vi "Offset_Loop_TS.vi"(0 "Port":u16, 1 "LV_Variables":T1={"ACQPS"=25, "Config_Enable"=1, "Prescale"=1, "ADC"=enum."A", "Adc_Channel"=1, "Ref_Int/EXT"=FALSE}, 2 "ACQPS":u16[](array[numeric]), 5 "Core":u16, 7 "Pin_Config":i32, 11 "error in":errorcluster, 12 "Voltage":dbl[](array[numeric]), 14 "VREF_Measured":dbl=2.5 format="%#_13g") -> (4 "Port Number out":u16, 6 "Core Number out":u16, 8 "output array":string[][](array[string]), 13 "OFF+GAIN":string[][](array[string]), 15 "error out":errorcluster)   [LabVIEW 2019]
uses:
  ADC_LV_Variables.ctl
  ADC_CTRL.ctl
  <userlib>/_TI-LA/Reusable/CCS/APIs/Data/Polymorphics/Write Data To Symbol - U16.vi
  <userlib>/_TI-LA/Reusable/CCS/APIs/CCS.lvlib
  <vilib>/Analysis/NI_AALBase.lvlib
  <userlib>/_TI-LA/Instr Drivers/Multimeter/Agilent 3446X Series/Agilent 3446X Series.lvlib
panel:
  out "AVG":dbl format="%0.2f"
  out "Array":dbl[](array[numeric])
  out "LV_Variables_out":T1={"ACQPS"=25, "Config_Enable"=1, "Prescale"=1, "ADC"=enum."A", "Adc_Channel"=1, "Ref_Int/EXT"=FALSE}
  in  "VISA_SGEN":refnum<visa-resource-name>="USB0::0x0957::0x1607::MY50001293::INSTR"
  out "standard deviation":dbl format="%0.2f"
  out "mean":dbl format="%0.2f"
  out "Waveform Graph":u16[](graph)
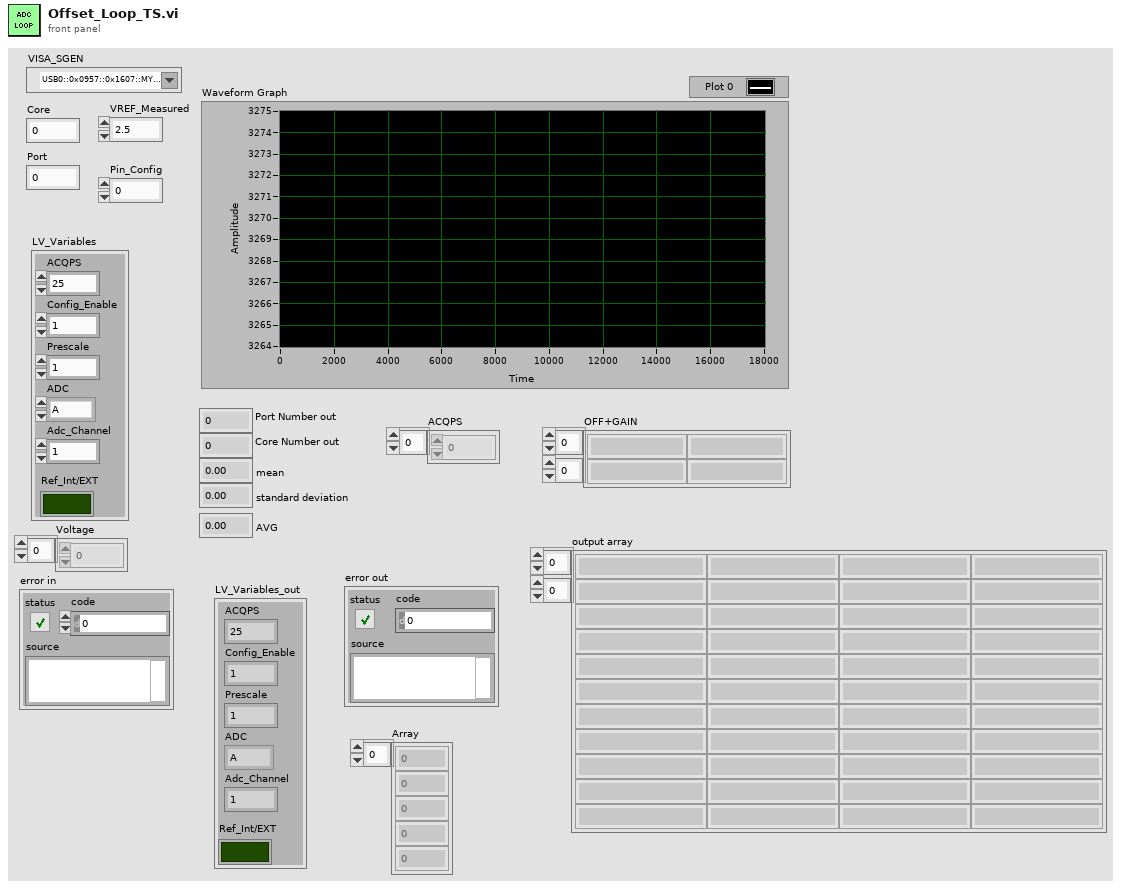
[diagram p1: front panel]
types:
  T1 = typedef "ADC_LV_Variables.ctl" = cluster{"ACQPS":u16, "Config_Enable":u16, "Prescale":u16, "ADC":T2, "Adc_Channel":u16, "Ref_Int/EXT":bool}
  T2 = typedef "ADC_CTRL.ctl" = enum16{"A", "B", "C"}
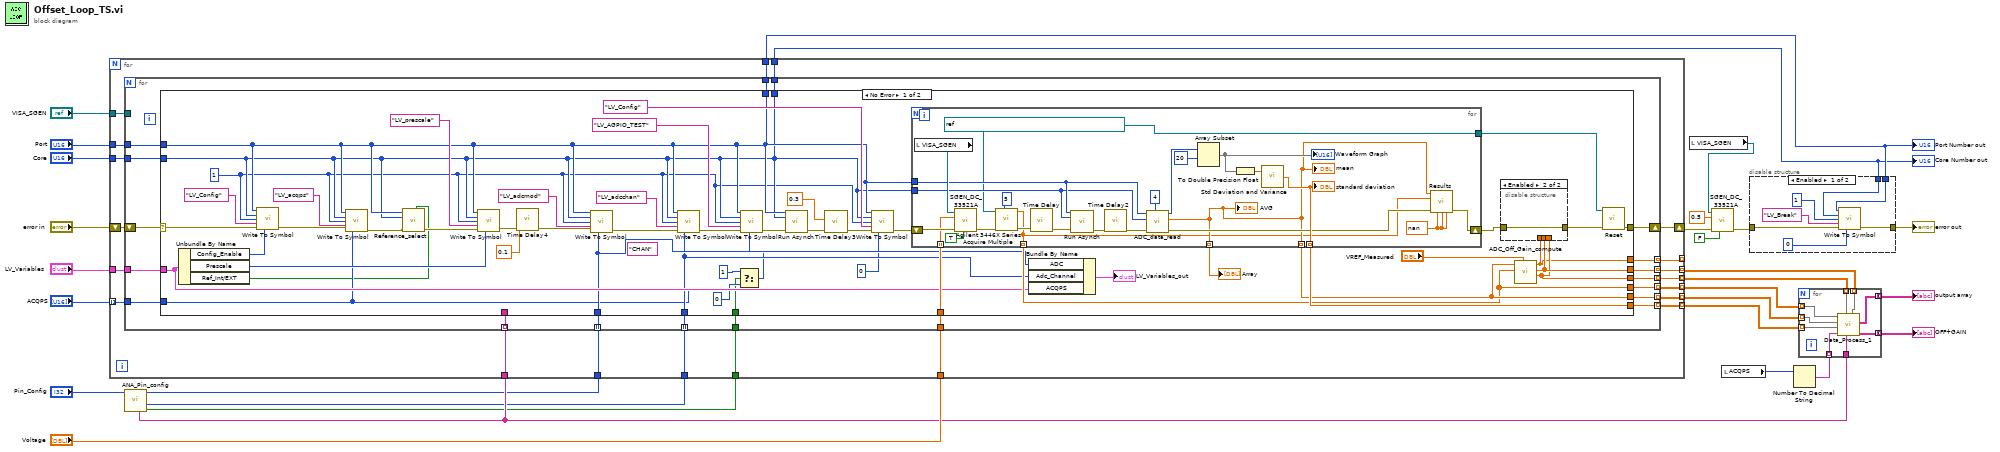
[diagram p0: block diagram]
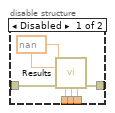
[diagram p3: hidden frame]
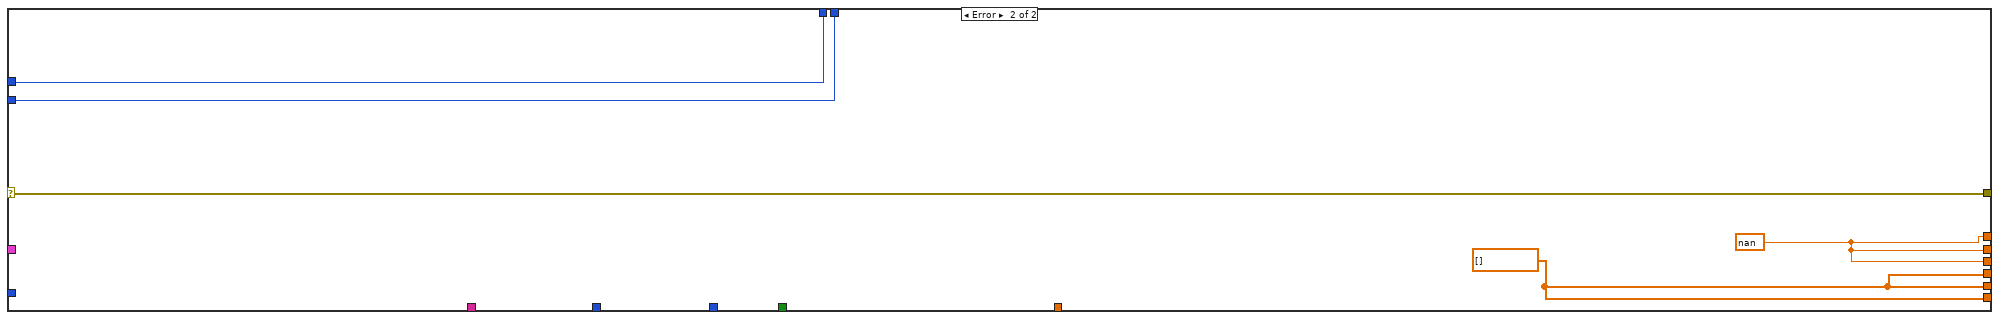
[diagram p4: hidden frame]
diagram:
  n1 = call "ANA_Pin_config.vi"("Pin_Config"="Pin_Config") -> ("Boolean"=w8:bool, "ADC_Channel"=w1:u16[], "ADC"=w2:T2[], "ADC+CH"=w9:string[])  [unwired: 7 in]
  n2 = for {
    tunnel: "Port" -> [w49]
    tunnel: "Core" -> [w48]
    tunnel: "LV_Variables" -> [w47]
    tunnel: [w45] -> w24
    tunnel: [w44] -> w23
    tunnel: w2 -> [w43]
    tunnel: w1 -> [w42]
    tunnel: "VISA_SGEN" -> [w41]
    tunnel: [w40] -> w10 mode=indexing
    tunnel: "Voltage" -> [w39]
    tunnel: [w38] -> w11 mode=indexing
    tunnel: [w37] -> w19 mode=indexing
    tunnel: [w36] -> w18 mode=indexing
    tunnel: [w35] -> w17 mode=indexing
    shift-right: [w46] -> w7
    shift-left: "error in" -> [w32]
    tunnel: "ACQPS" -> [w34] mode=indexing
    tunnel: w9 -> [w33]
    tunnel: w8 -> [w31]
    tunnel: [w30] -> _ mode=indexing
    n3 = for {
      tunnel: w49 -> [w65]
      tunnel: w48 -> [w66]
      tunnel: w47 -> [w67]
      shift-right: [w68] -> w46
      shift-left: w32 -> [w62]
      tunnel: [w63] -> w44
      tunnel: [w64] -> w45
      tunnel: w43 -> [w54] mode=indexing
      tunnel: w42 -> [w61] mode=indexing
      tunnel: [w60] -> w36 mode=indexing
      tunnel: [w59] -> w35 mode=indexing
      tunnel: w39 -> [w58]
      tunnel: w41 -> [_]
      tunnel: [w57] -> w40 mode=indexing
      tunnel: [w56] -> w38 mode=indexing
      tunnel: [w55] -> w37 mode=indexing
      tunnel: w34 -> [w53]
      tunnel: w33 -> [w52] mode=indexing
      tunnel: w31 -> [w51]
      tunnel: [w50] -> w30 mode=indexing
      n4 = case shown="No Error" w62 {
        selector: w62 -> [w111 w152]
        tunnel: [w92 w152] -> w68
        tunnel: w67 -> [w105 _]
        tunnel: w65 -> [w79 w154]
        tunnel: w66 -> [w78 w153]
        tunnel: [w79 w154] -> w64
        tunnel: [w78 w153] -> w63
        tunnel: w61 -> [w102 _]
        tunnel: [w109 w151] -> w60
        tunnel: [w110 w151] -> w59
        tunnel: w58 -> [w108 _]
        tunnel: [w89 w150] -> w57
        tunnel: [w88 w150] -> w56
        tunnel: [w107 w151] -> w55
        tunnel: w54 -> [w103 _]
        tunnel: w53 -> [w72 _]
        tunnel: w52 -> [_ _]
        tunnel: w51 -> [w95 _]
        tunnel: [w70 w150] -> w50
        frame No Error {
          (unwired) "CHAN" ("Name")
          w77 = 1 ("Page")
          n5 = Unbundle By Name(w105) -> ("Config_Enable"=w114:u16, "Prescale"=w106:u16, "Ref_Int/EXT"=w69:bool)
          n6 = call-poly <userlib>:"Write To Symbol.vi"("Port Number"=w79, "Core Number"=w78, "Page"=w77, "Symbol Name"="LV_Config", "error in"=w111, "Write Data"=w114) -> ("error out"=w118:errorcluster)  [unwired: 7 in, 2 out]
          n7 = call-poly <userlib>:"Write To Symbol.vi"("Port Number"=w79, "Core Number"=w78, "Page"=w77, "Symbol Name"="LV_acqps", "error in"=w118, "Write Data"=w72) -> ("error out"=w94:errorcluster)  [unwired: 7 in, 2 out]
          n8 = call "Reference_select.vi"("Internal_Ref"=w69, "error in"=w94, "Core Number"=w78, "Port Number"=w79) -> ("error out"=w93:errorcluster)  [unwired: 7 in]
          n9 = call-poly <userlib>:"Write To Symbol.vi"("Port Number"=w79, "Core Number"=w78, "Page"=w77, "Symbol Name"="LV_prescale", "error in"=w93, "Write Data"=w106) -> ("error out"=w76:errorcluster)  [unwired: 7 in, 2 out]
          n10 = call "Time Delay4"("error in (no error)"=w76, "Delay Time (s)"=0.1) -> ("error out"=w75:errorcluster)  [unwired: 9 in]
          n11 = call-poly <userlib>:"Write To Symbol.vi"("Port Number"=w79, "Core Number"=w78, "Page"=w77, "Symbol Name"="LV_adcmod", "error in"=w75, "Write Data"=w103) -> ("error out"=w101:errorcluster)  [unwired: 7 in, 2 out]
          n12 = call-poly <userlib>:"Write To Symbol.vi"("Port Number"=w79, "Core Number"=w78, "Page"=w77, "Symbol Name"="LV_adcchan", "error in"=w101, "Write Data"=w102) -> ("error out"=w100:errorcluster)  [unwired: 7 in, 2 out]
          n13 = Select(t=u16 1, s=w95, f=u16 0) -> (s? t:f=w98:u16)
          n14 = call-poly <userlib>:"Write To Symbol.vi"("Port Number"=w79, "Core Number"=w78, "Page"=w77, "Symbol Name"="LV_AGPIO_TEST", "error in"=w100, "Write Data"=w98) -> ("error out"=w85:errorcluster)  [unwired: 7 in, 2 out]
          n15 = call <userlib>:"Run Asynch.vi"("Port Number"=w79, "Core Number"=w78, "error in"=w85) -> ("error out"=w73:errorcluster)  [unwired: 10 in, 2 out]
          n16 = call "Time Delay3"("error in (no error)"=w73, "Delay Time (s)"=0.3) -> ("error out"=w83:errorcluster)  [unwired: 9 in]
          n17 = call-poly <userlib>:"Write To Symbol.vi"("Port Number"=w79, "Core Number"=w78, "Page"=w77, "Symbol Name"="LV_Config", "error in"=w83, "Write Data"=u16 0) -> ("error out"=w82:errorcluster)  [unwired: 7 in, 2 out]
          n18 = for {
            tunnel: w79 -> [w138]
            tunnel: w78 -> [w137]
            tunnel: [w127] -> w109 mode=indexing
            tunnel: [w144] -> w110 mode=indexing
            shift-right: [w130] -> w90
            shift-left: w82 -> [w141]
            tunnel: w108 -> [w136] mode=indexing
            tunnel: [w126] -> w107 mode=indexing
            tunnel: [w132] -> w91
            tunnel: [w127] -> w87 mode=indexing
            w129 = nan
            w132 = refnum<visa-resource-name> "USB0::0x2A8D::0x1301::MY57222838::INSTR" ("VISA resource name")
            n19 = local read "VISA_SGEN"() -> (w143:refnum<visa-resource-name>)
            n20 = call "SGEN_DC_33521A.vi"("Enable Output (T: Enable)"=TRUE, "error in (no error)"=w141, "DC Offset (0 V)"=w136, "VISA_SGEN"=w143) -> ("error out"=w135:errorcluster)  [unwired: 7 in]
            n21 = call "Agilent 3446X Series Acquire Multiple.vi"("Sample Count (1)"=5, "error in (no error)"=w135, "VISA resource name"=w132) -> ("error out"=w134:errorcluster, "mean"=w126:dbl)  [unwired: 6 in, 1 out]
            n22 = call "Time Delay"("error in (no error)"=w134) -> ("error out"=w142:errorcluster)  [unwired: 10 in]
            n23 = call <userlib>:"Run Asynch.vi"("Port Number"=w138, "Core Number"=w137, "error in"=w142) -> ("error out"=w140:errorcluster)  [unwired: 10 in, 2 out]
            n24 = call "Time Delay2"("error in (no error)"=w140) -> ("error out"=w139:errorcluster)  [unwired: 10 in]
            n25 = call "ADC_data_read.vi"("No_Iterations"=4, "error in (no error)"=w139, "Core Number"=w137, "Port Number"=w138) -> ("error out"=w131:errorcluster, "Read Data"=w127:dbl, "Read Data[]"=w146:u16[])  [unwired: 5 in]
            "mean" <- w127
            "AVG" <- w127
            n26 = Array Subset(array=w146, index=20) -> (w145:u16[])  [unwired: 1 in]
            "Waveform Graph" <- w145
            n27 = To Double Precision Float(number=w145) -> (double precision float=w148:dbl[])
            n28 = call <vilib>:"Std Deviation and Variance.vi"("X"=w148) -> ("standard deviation"=w144:dbl)  [unwired: 1 in, 2 out]
            "standard deviation" <- w144
            n29 = call "Results.vi"("Code"=w127, "Voltage"=w126, "Error In"=w131, "Slope"=w129, "Offset_Error"=w129, "Gain_error"=w129) -> ("error out"=w130:errorcluster)  [unwired: 9 in]
          }
          "Array" <- w87
          n30 = Bundle By Name(cluster=w105, "ADC"=w103, "Adc_Channel"=w102, "ACQPS"=w72) -> (→"LV_Variables_out":T1)
          n31 = call "ADC_Off_Gain_compute.vi"("VREF_Measured"="VREF_Measured", "Voltage_Array"=w107, "Code"=w109) -> ("Gain_Error_(LSB)"=w88:dbl, "Offset_Error"=w89:dbl, "slope"=w70:dbl)  [unwired: 5 in, 1 out]
          n32 = disable-structure shown="Enabled" {
            disable-tunnel: w90 -> [w124 w125]
            disable-tunnel: w70 -> [w122 _]
            disable-tunnel: w89 -> [w121 _]
            disable-tunnel: w88 -> [w120 _]
            disable-tunnel: [w119 w125] -> w71
            frame Disabled {
              w123 = nan
              n33 = call "Results.vi"("Code"=w123, "Voltage"=w123, "Error In"=w124, "Slope"=w122, "Offset_Error"=w121, "Gain_error"=w120) -> ("error out"=w119:errorcluster)  [unwired: 9 in]
            }
            frame Enabled {
            }
          }
          n34 = call <userlib>:"Reset.vi"("error in (no error)"=w71, "VISA resource name"=w91) -> ("error out"=w92:errorcluster)  [unwired: 8 in, 1 out]
        }
        frame Error {
          w150 = nan
          w151 = dbl[] []
        }
      }
    }
  }
  "Core Number out" <- w23
  "Port Number out" <- w24
  n35 = local read "VISA_SGEN"() -> (w5:refnum<visa-resource-name>)
  n36 = call "SGEN_DC_33521A.vi"("Enable Output (T: Enable)"=FALSE, "error in (no error)"=w7, "DC Offset (0 V)"=0.5, "VISA_SGEN"=w5) -> ("error out"=w6:errorcluster)  [unwired: 7 in]
  n37 = local read "ACQPS"() -> (w14:u16[])
  n38 = disable-structure shown="Enabled" {
    disable-tunnel: w6 -> [w158 w162]
    disable-tunnel: [w155 w162] -> w25
    disable-tunnel: w24 -> [w157 _]
    disable-tunnel: w23 -> [w156 _]
    frame Enabled {
      n39 = call-poly <userlib>:"Write To Symbol.vi"("Port Number"=w157, "Core Number"=w156, "Page"=1, "Symbol Name"="LV_Break", "error in"=w158, "Write Data"=u16 0) -> ("error out"=w155:errorcluster)  [unwired: 7 in, 2 out]
    }
    frame Disabled {
    }
  }
  "error out" <- w25
  n40 = Number To Decimal String(number=w14) -> (decimal integer string=w13:string[])  [unwired: 1 in]
  n41 = for {
    tunnel: w19 -> [w171] mode=indexing
    tunnel: w18 -> [w170] mode=indexing
    tunnel: w17 -> [w169] mode=indexing
    tunnel: w9 -> [w168]
    tunnel: w13 -> [w167] mode=indexing
    tunnel: [w166] -> w15 mode=concatenating
    tunnel: [w165] -> w12 mode=concatenating
    tunnel: w11 -> [w164] mode=indexing
    tunnel: w10 -> [w163] mode=indexing
    n42 = call "Data_Process_1.vi"("Offset_Error"=w163, "ADC+CH"=w168, "Gain_Error"=w164, "ACQPS"=w167, "Std_Deviation"=w169, "Mean"=w170, "Vin_Measured"=w171) -> ("OFF+GAIN"=w165:string[][], "output array"=w166:string[][])  [unwired: 3 in]
  }
  "output array" <- w15
  "OFF+GAIN" <- w12
